vi "Read Messages.vi"(8 "error in":errorcluster, 11 "channel ref in":refnum<k20>) -> (0 "error out":errorcluster, 2 "messages":T1[](array[typedef]), 3 "channel ref out":refnum<k20>)   [LabVIEW 2020, in "MIL-STD 1553 Import.lvlib"]
uses:
  MIL-STD 1553 Import.lvlib
  6771c8a3-f311-47c1-9371-f84e0ba0f73c.vi
  Constants.vi
  3f34854b-cbb0-4767-be42-acd70d4bd91c.vi
  Shared/Message Type.ctl
  Shared/Address.ctl
  Shared/Terminal Endpoint.ctl
  Shared/Parameter Definition.ctl
  Shared/Message Definition.ctl
  d9ed25fc-d4e2-449f-a9ba-1571765a02e2.vi
  5b48f9ba-a688-4834-891e-a2f49df4034f.vi
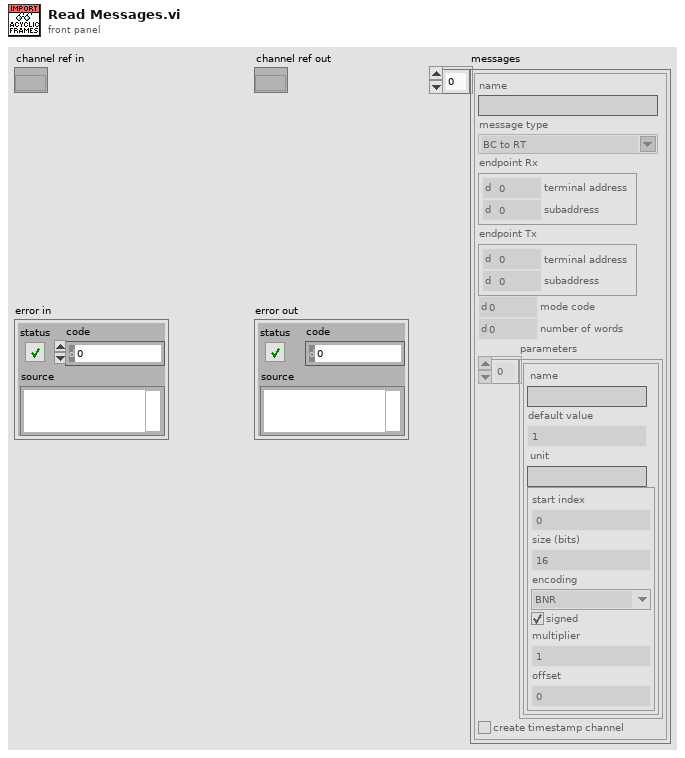
[diagram p1: front panel]
types:
  T1 = typedef "Message Definition.ctl" = cluster{"name":string, "message type":T2, "endpoint Rx":T3, "endpoint Tx":T3, "mode code":u16, "number of words":u16, "parameters":cluster{"name":string, "default value":dbl, "unit":string, "parameter definition":T5}[], "create timestamp channel":bool}
  T2 = typedef "Message Type.ctl" = string
  T3 = typedef "Terminal Endpoint.ctl" = cluster{"terminal address":T4, "subaddress":T4}
  T4 = typedef "Address.ctl" = u16
  T5 = typedef "Parameter Definition.ctl" = cluster{"start index":i32, "size (bits)":i32, "encoding":enum16{"BNR", "BCD", "Discrete"}, "signed":bool, "multiplier":dbl, "offset":dbl}
  T6 = cluster{"name":string, "default value":dbl, "unit":string, "parameter definition":T5}[]
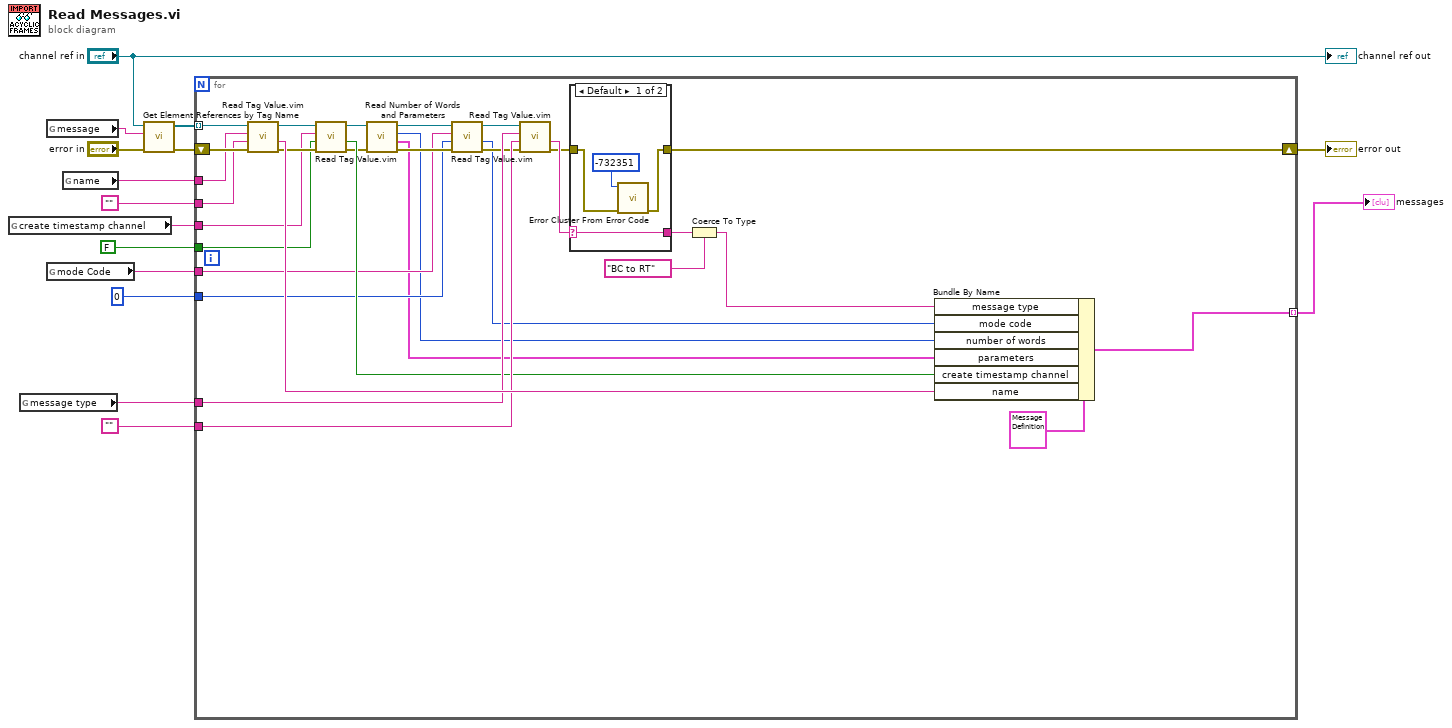
[diagram p0: block diagram]
diagram:
  n1 = global read "Constants.vi" "create timestamp channel"() -> (w4:string)
  n2 = global read "Constants.vi" "message type"() -> (w7:string)
  n3 = global read "Constants.vi" "message"() -> (w15:string)
  n4 = global read "Constants.vi" "mode Code"() -> (w2:string)
  n5 = global read "Constants.vi" "name"() -> (w10:string)
  n6 = call "Get Element References by Tag Name.vi"("error in"="error in", "tag name"=w15, "node in"="channel ref in") -> ("error out"=w12:errorcluster, "array of elements"=w14:refnum<k20>[])  [unwired: 7 in]
  n7 = for {
    shift-right: [w33] -> w13
    shift-left: w12 -> [w46]
    tunnel: w14 -> [w45] mode=indexing
    tunnel: w10 -> [w44]
    tunnel: "" -> [w43]
    tunnel: w7 -> [w40]
    tunnel: "" -> [w39]
    tunnel: [w32] -> w5 mode=indexing
    tunnel: w4 -> [w29]
    tunnel: FALSE -> [w28]
    tunnel: w2 -> [w20]
    tunnel: u16 0 -> [w19]
    n8 = call "Read Tag Value.vim"("error in"=w46, "default"=w43, "tag name"=w44, "node in"=w45) -> ("error out"=w30:errorcluster, "value"=w41:string, "node out"=w31:refnum<k20>)  [unwired: 5 in]
    n9 = call "Read Tag Value.vim"("error in"=w30, "default"=w28, "tag name"=w29, "node in"=w31) -> ("error out"=w25:errorcluster, "value"=w27:bool, "node out"=w26:refnum<k20>)  [unwired: 5 in]
    n10 = call "Read Number of Words and Parameters.vi"("error in"=w25, "message ref in"=w26) -> ("error out"=w23:errorcluster, "parameters"=w16:T6, "number of words"=w18:u16, "message ref out"=w24:refnum<k20>)  [unwired: 6 in]
    n11 = call "Read Tag Value.vim"("error in"=w23, "default"=w19, "tag name"=w20, "node in"=w24) -> ("error out"=w21:errorcluster, "value"=w17:u16, "node out"=w22:refnum<k20>)  [unwired: 5 in]
    n12 = call "Read Tag Value.vim"("error in"=w21, "default"=w39, "tag name"=w40, "node in"=w22) -> ("error out"=w37:errorcluster, "value"=w38:string)  [unwired: 5 in, 1 out]
    n13 = case shown="Default" w38 {
      selector: w38 -> [w50 w51]
      tunnel: [w48 w52] -> w33
      tunnel: w37 -> [w49 w52]
      tunnel: [w50 w51] -> w35
      frame Default {
        n14 = call <vilib>:"Error Cluster From Error Code.vi"("error in (no error)"=w49, "error code (0)"=-732351) -> ("error out"=w48:errorcluster)  [unwired: 7 in]
      }
      frame "BC to RT", "MC", "RT to BC", "RT to RT" {
      }
    }
    n15 = Coerce To Type(0:w35, 1:T2 "BC to RT" ("message type")) -> (2:w34:T2)
    n16 = Bundle By Name(cluster=T1 {"name"="", "message type"="BC to RT", "endpoint Rx"={"terminal address"=0, "subaddress"=0}, "endpoint Tx"={"terminal address"=0, "subaddress"=0}, "mode code"=0, "number of words"=0, "parameters"=[], "create timestamp channel"=FALSE} ("message definition"), "message type"=w34, "mode code"=w17, "number of words"=w18, "parameters"=w16, "create timestamp channel"=w27, "name"=w41) -> (w32:T1)
  }
  "error out" <- w13
  "messages" <- w5
  "channel ref out" <- "channel ref in"
